vi "FGA Feed Watchdog.vi"(1 "Watchdog Dish":T1) -> (0 "Watchdog Fed?":bool)   [LabVIEW 2009]
uses:
  UI Comm/Watchdog Dish Labels.ctl
  Actions for FG's.ctl
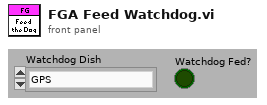
[diagram p1: front panel]
types:
  T1 = typedef "Watchdog Dish Labels.ctl" = enum16{"GPS", "SICK", "Compass", "Cameras", "Motor Controller", "Debug", "RC Receiver"}
  T2 = typedef "Actions for FG's.ctl" = enum16{"Read", "Write"}
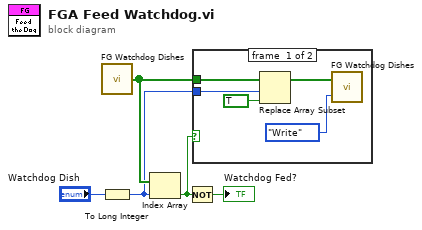
[diagram p0: block diagram]
diagram:
  n1 = call "FG Watchdog Dishes.vi"() -> ("Watchdog dishes out"=w4:bool[])  [unwired: 2 in]
  n2 = To Long Integer(number="Watchdog Dish") -> (32bit integer=w3:i32)
  n3 = Index Array(array=w4, index=w3) -> (element=w1:bool)
  n4 = Not(x=w1) -> (.not. x?=→"Watchdog Fed?":bool)
  n5 = case shown="False" w1 {
    tunnel: w4 -> [w10 _]
    tunnel: w3 -> [w9 _]
    frame #0 {
      n6 = Replace Array Subset(array=w10, new element=TRUE ("new element/subarray"), index=w9) -> (w7:bool[])
      n7 = call "FG Watchdog Dishes.vi"("FG Action (Read)"=Actions_for_FG's."Write", "Watchdog dishes in"=w7) -> ()  [unwired: 1 out]
    }
    frame #1 {
    }
  }
